vi "Read from Excel file.vi"(7 "sheetname (\"\") - leave blank for first sheet":string, 8 "error in (no error)":errorcluster, 11 "File Name":path=path "C:/PhaeronGit/LVNPOI/Scratch/test.xls") -> (0 "error out":errorcluster, 2 "Values":string[][](array[string]))   [LabVIEW 2014]
doc: "Writes the 2D string array to the named Excel format file."
uses:
  Data/Polymorphic VIs/Get Cells (2D Row Part String).vi
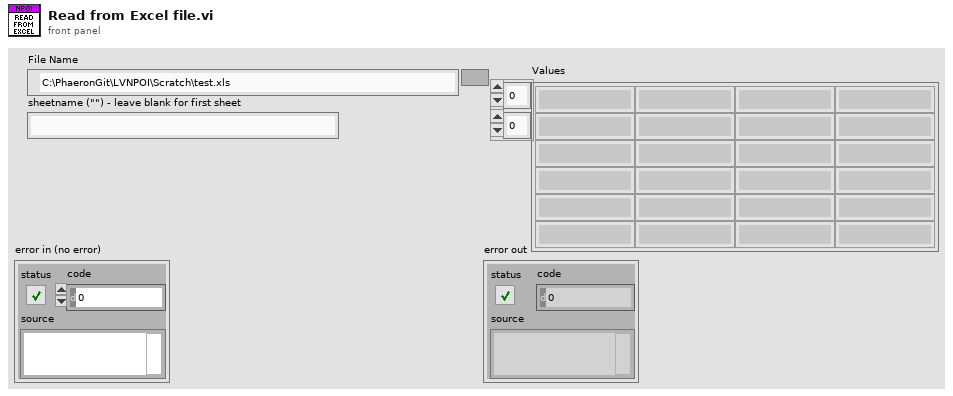
[diagram p1: front panel]
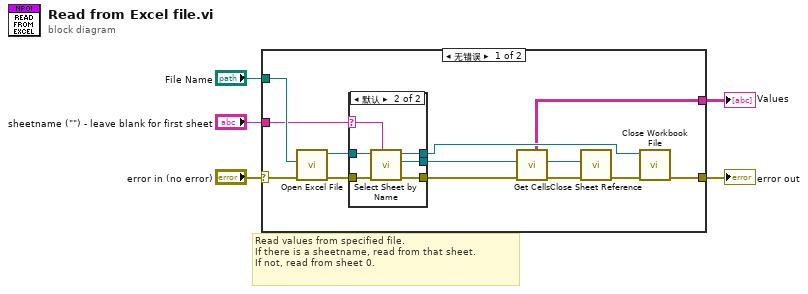
[diagram p0: block diagram]
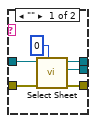
[diagram p2: hidden frame]
diagram:
  # "Read values from specified file.\nIf there is a sheetname, read from that sheet.\nIf not, read from sheet 0."
  n1 = case shown="无错误" "error in (no error)" {
    selector: "error in (no error)" -> [w17 w31]
    tunnel: "File Name" -> [w16 _]
    tunnel: "sheetname (\"\") - leave blank for first sheet" -> [w13 _]
    tunnel: [w18 w31] -> w3
    tunnel: [w6 _] -> w1
    frame No Error {
      n2 = call "Open Excel File.vi"("error in (no error)"=w17, "File Name"=w16) -> ("error out"=w15:errorcluster, "IWorkbook Reference Out"=w14:refnum<k24>)  [unwired: 8 in]
      n3 = case shown="默认" w13 {
        selector: w13 -> [_ w28]
        tunnel: w15 -> [w24 w30]
        tunnel: w14 -> [w23 w29]
        tunnel: [w21 w27] -> w7
        tunnel: [w20 w26] -> w11
        tunnel: [w19 w25] -> w12
        frame "" {
          n4 = call "Select Sheet.vi"("Sheet (0)"=0 ("Sheet"), "error in (no error)"=w24, "IWorkbook Reference"=w23) -> ("error out"=w19:errorcluster, "Sheet Reference"=w20:refnum<k24>, "IWorkbook Reference"=w21:refnum<k24>)  [unwired: 6 in]
        }
        frame Default {
          n5 = call "Select Sheet by Name.vi"("Sheet (Sheet1)"=w28, "error in (no error)"=w30, "IWorkbook Reference"=w29) -> ("error out"=w25:errorcluster, "Sheet Reference"=w26:refnum<k24>, "IWorkbook Reference"=w27:refnum<k24>)  [unwired: 6 in]
        }
      }
      n6 = call-poly "Get Cells.vi"("error in (no error)"=w12, "Sheet Reference"=w11) -> ("error out"=w10:errorcluster, "Sheet Reference out"=w9:refnum<k24>, "Values"=w6:string[][])  [unwired: 7 in]
      n7 = call "Close Sheet Reference.vi"("error in (no error)"=w10, "Sheet Reference"=w9) -> ("error out"=w8:errorcluster)  [unwired: 9 in]
      n8 = call "Close Workbook File.vi"("error in (no error)"=w8, "IWorkbook Reference"=w7) -> ("error out"=w18:errorcluster)  [unwired: 9 in]
    }
    frame Error {
    }
  }
  "error out" <- w3
  "Values" <- w1
